vi "Oclaro_FB_INJ_ActiveSampling.vi"(1 "Resistance (k Ohms)":dbl=10.0) -> ()   [LabVIEW 2014]
doc: "Use this template to measure or generate signals using the DAQ Assistant Express VI and NI-DAQmx. Double click the DAQ Assistant Express VI to launch a configuration wizard which steps you through configuring a measurement or generation.\n\nNote: You must have an NI-DAQmx compatible device installed to use this Express VI. Refer to the DAQ Quick Start Guide for NI-DAQ 7.0 for a list of compatible devices."
uses:
  <vilib>/addons/zeromq/socket_type.ctl
  Instance           8 18Saved   INJ FB Map .vi
  <instrlib>/Tektronix 7000 Series/Public/Data/Read (Single Waveform).vi
  <instrlib>/Tektronix 7000 Series/Tektronix 7000 Series.lvlib
  <vilib>/addons/zeromq/zeromq.lvlib
  <vilib>/addons/zeromq/zmq_context.lvclass
  <vilib>/addons/zeromq/zmq_socket.lvclass
panel:
  in  "AOM Channel":bool
  out "Status":string="Complete"
  out "Start time":timestamp=timestamp(3523998390.26649 s since 1904-01-01)
  in  "Current Source Address":refnum<visa-resource-name>="GPIB0::3::INSTR"
  in  "TEC Address":refnum<visa-resource-name>="GPIB0::3::INSTR"
  in  "Channel (0: Channel 1)":u16(ring)=3 format="%#_5f" items=["Channel 1", "Channel 2", "Channel 3", "Channel 4", "Math 1", "Math 2", "Math 3", "Math 4", "Reference 1", "Reference 2", "Reference 3", "Reference 4"]
  out "Total Time (hrs)":dbl=0.15259278178215027
  out "Finish time":timestamp=timestamp(3523998939.6005044 s since 1904-01-01)
  in  "Tek Scope Address":refnum<visa-resource-name>="GPIB0::4::INSTR"
  in  "Time to wait for TEC (sec)":dbl=10.0 caption="Delay Time (s)"
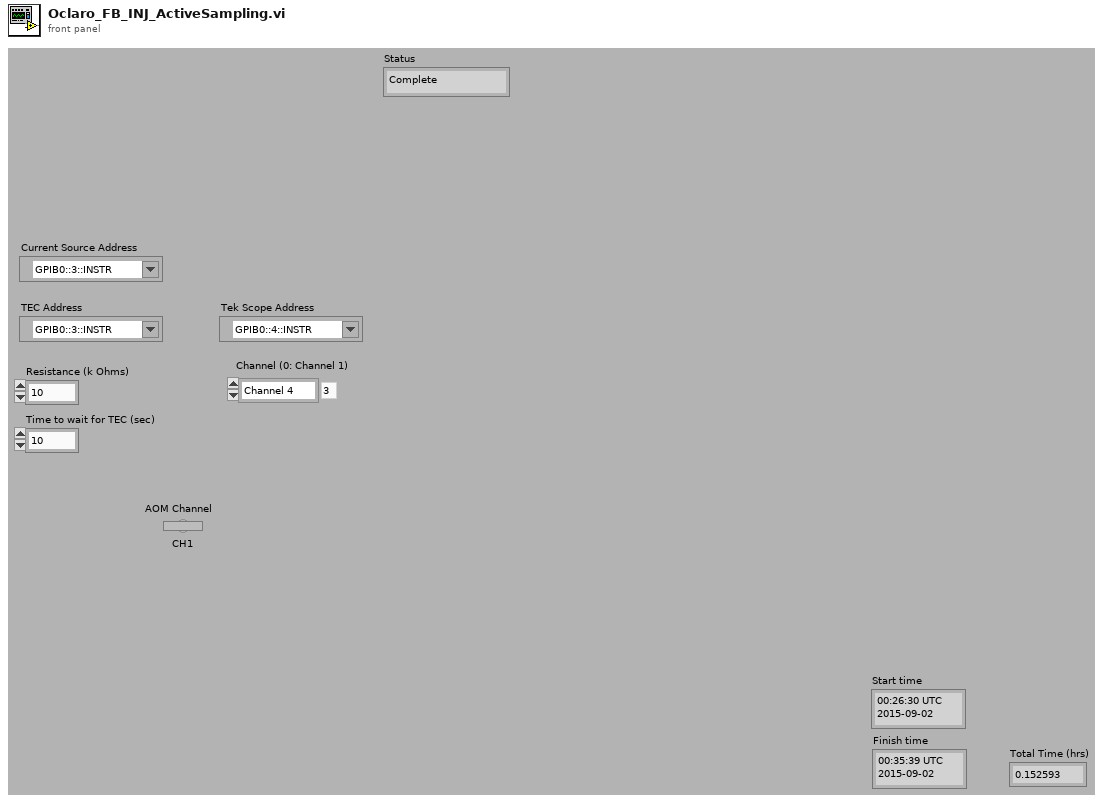
[diagram p1: front panel]
types:
  T1 = typedef "zeromq.lvlib/socket_type.ctl" = enum8{"ZMQ_PAIR", "ZMQ_PUB", "ZMQ_SUB", "ZMQ_REQ", "ZMQ_REP", "ZMQ_DEALER", "ZMQ_ROUTER", "ZMQ_PULL", "ZMQ_PUSH", "ZMQ_XPUB", "ZMQ_XSUB"}
  T2 = enum16{"big-endian, network order", "native, host order", "little-endian"}
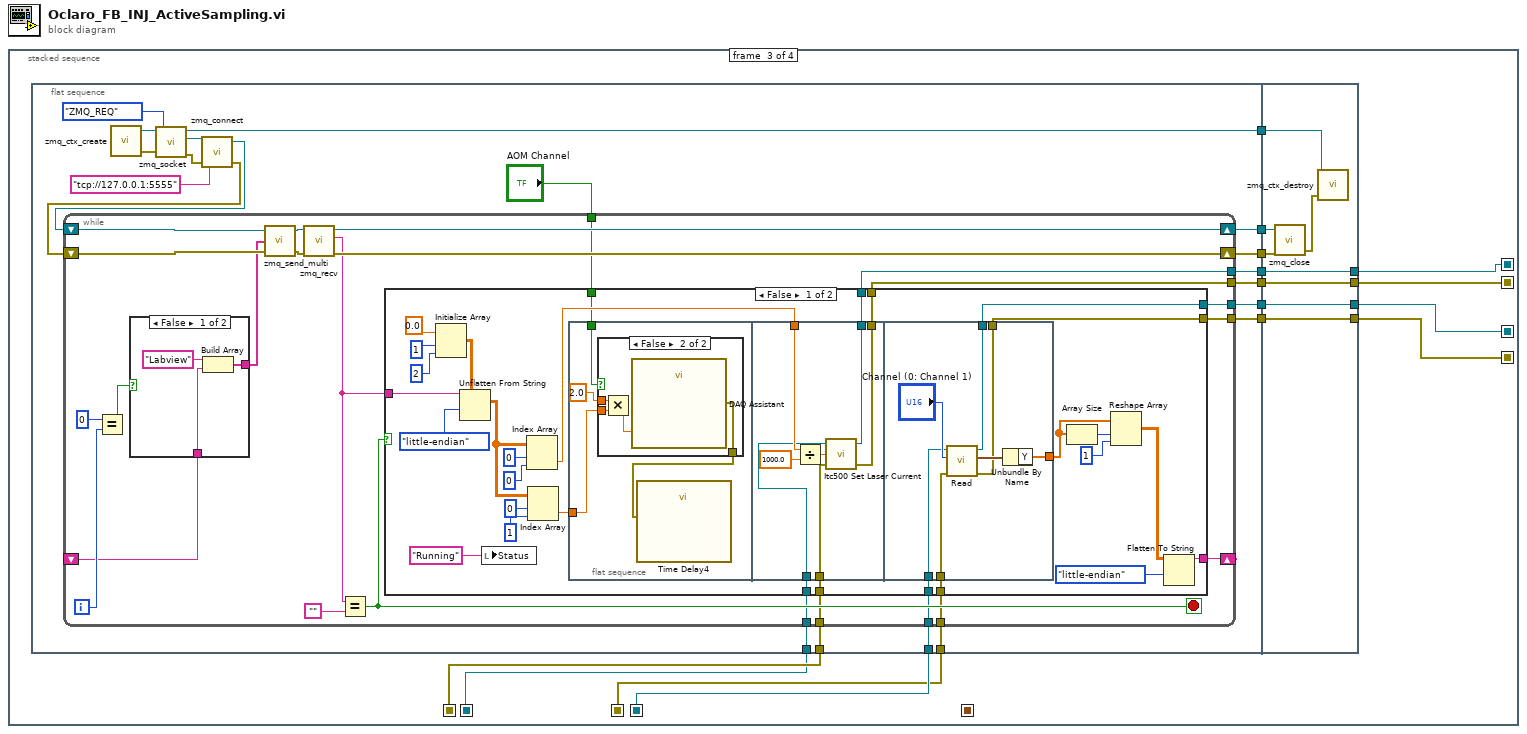
[diagram p0: block diagram]
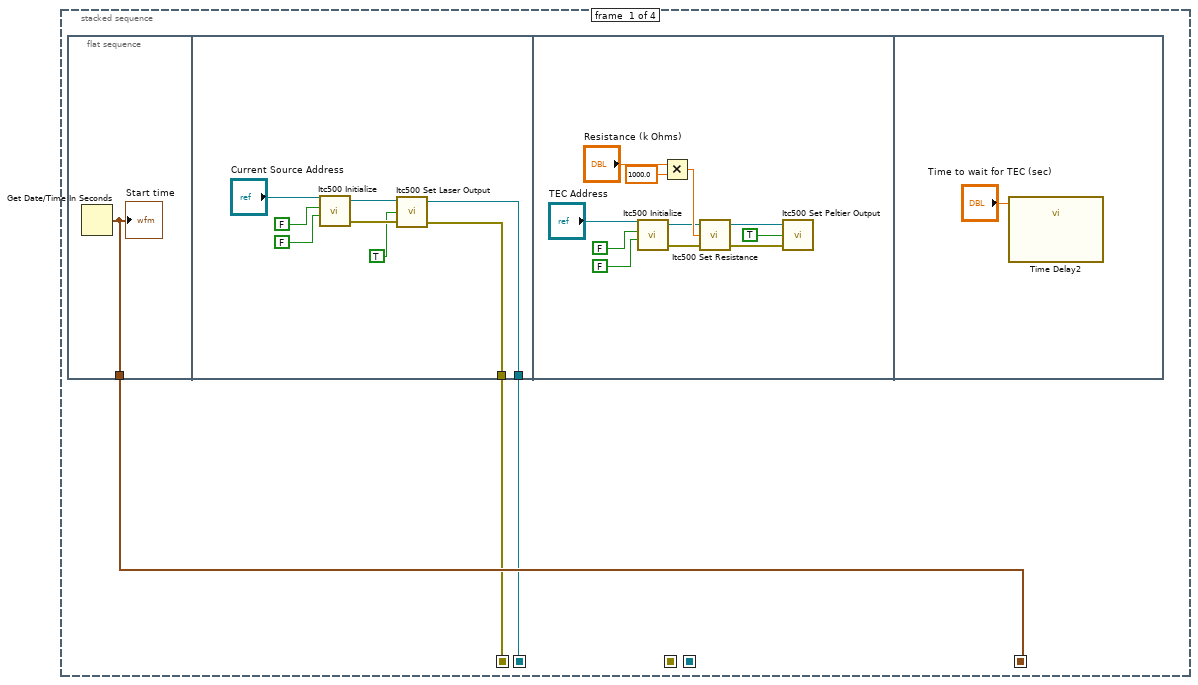
[diagram p2: hidden frame]
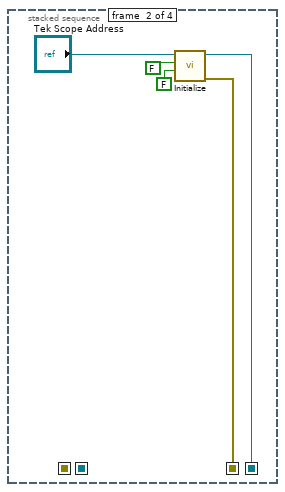
[diagram p3: hidden frame]
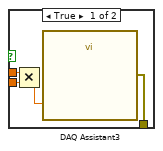
[diagram p4: hidden frame]
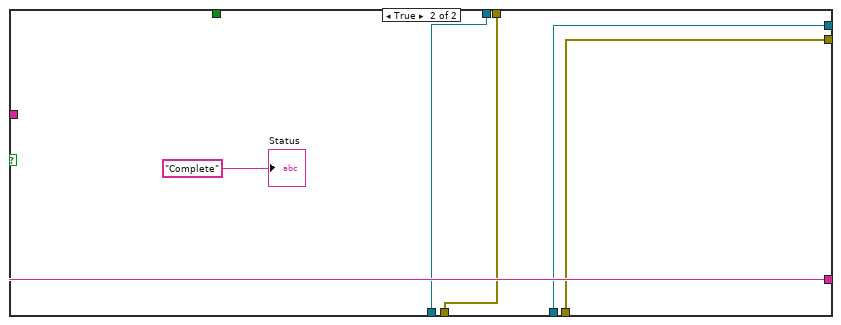
[diagram p5: hidden frame]
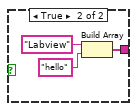
[diagram p6: hidden frame]
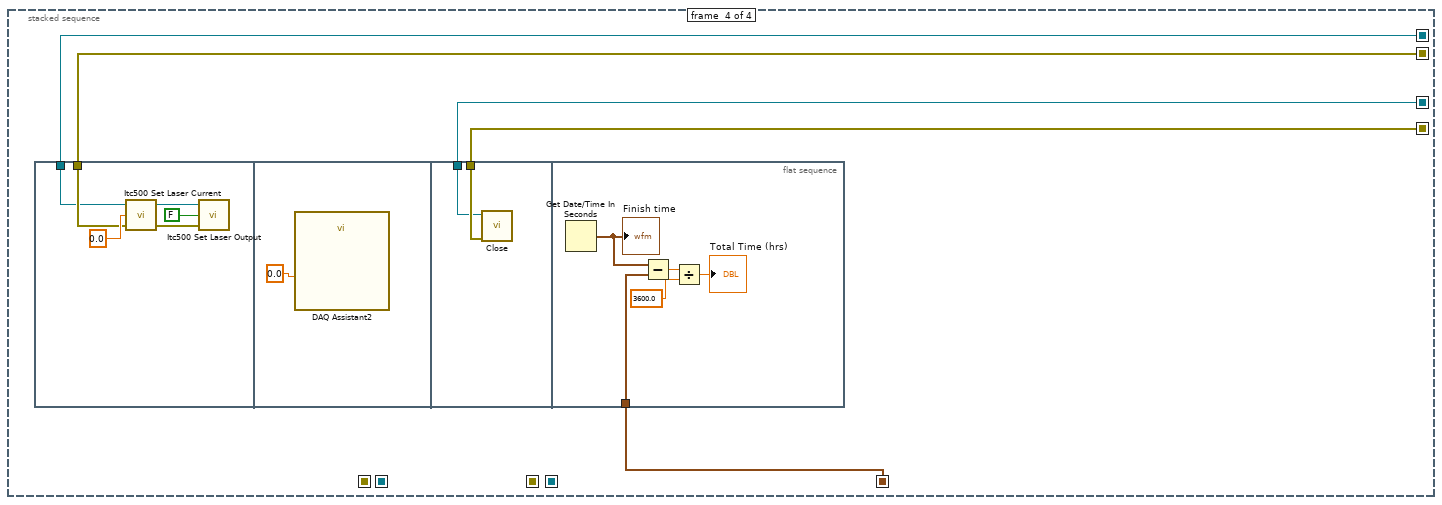
[diagram p7: hidden frame]
diagram:
  n1 = stacked-sequence {
    seq-local: [_ w25 _ _] -> [_ _ w38 _]
    seq-local: [_ w26 _ _] -> [_ _ w39 _]
    seq-local: [_ _ w30 _] -> [_ _ _ w167]
    seq-local: [_ _ w32 _] -> [_ _ _ w168]
    seq-local: [w3 _ _ _] -> [_ _ _ w164]
    seq-local: [_ _ w34 _] -> [_ _ _ w165]
    seq-local: [_ _ w36 _] -> [_ _ _ w166]
    seq-local: [w1 _ _ _] -> [_ _ w40 _]
    seq-local: [w2 _ _ _] -> [_ _ w41 _]
    frame #0 {
      n2 = flat-sequence {
        tunnel: [w4] -> w3
        tunnel: [w6] -> w2
        tunnel: [w5] -> w1
        frame #0 {
          n3 = Get Date/Time In Seconds() -> (seconds since 1Jan1904=w4:timestamp)
          "Start time" <- w4
        }
        frame #1 {
          n4 = call <instrlib>:"Itc500 Initialize.vi"("reset device"=FALSE, "id query"=FALSE, "resource name"="Current Source Address") -> ("error out"=w12:errorcluster, "instrument handle"=w11:refnum<visa-resource-name>)  [unwired: 1 in, 1 out]
          n5 = call <instrlib>:"Itc500 Set Laser Output.vi"("error in (no error)"=w12, "output"=TRUE, "instrument handle"=w11) -> ("error out"=w6:errorcluster, "instrument handle out"=w5:refnum<visa-resource-name>)  [unwired: 1 out]
        }
        frame #2 {
          n6 = call <instrlib>:"Itc500 Initialize.vi"("reset device"=FALSE, "id query"=FALSE, "resource name"="TEC Address") -> ("error out"=w19:errorcluster, "instrument handle"=w18:refnum<visa-resource-name>)  [unwired: 1 in, 1 out]
          n7 = Multiply(x="Resistance (k Ohms)", y=1000.0) -> (x*y=w22:dbl)
          n8 = call <instrlib>:"Itc500 Set Resistance.vi"("error in (no error)"=w19, "resistance"=w22, "instrument handle"=w18) -> ("error out"=w16:errorcluster, "instrument handle out"=w15:refnum<visa-resource-name>)  [unwired: 1 out]
          n9 = call <instrlib>:"Itc500 Set Peltier Output.vi"("error in (no error)"=w16, "output"=TRUE, "instrument handle"=w15) -> ()  [unwired: 3 out]
        }
        frame #3 {
          n10 = call "Time Delay2"("Delay Time (s)"="Time to wait for TEC (sec)") -> ()  [unwired: 10 in, 1 out]
        }
      }
    }
    frame #1 {
      n11 = call <instrlib>:"Initialize.vi"("Reset? ( Yes)"=FALSE ("Reset (T: Reset)"), "ID Query? ( Yes)"=FALSE ("Reset (T: Reset)"), "VISA resource name"="Tek Scope Address") -> ("error out"=w25:errorcluster, "VISA resource name out"=w26:refnum<visa-resource-name>)  [unwired: 7 in]
    }
    frame #2 {
      n12 = flat-sequence {
        tunnel: [w60] -> w44
        tunnel: [w54] -> w43
        tunnel: [w55] -> w42
        tunnel: w41 -> [w53]
        tunnel: w40 -> [w52]
        tunnel: w39 -> [w51]
        tunnel: w38 -> [w50]
        tunnel: [w49] -> w37
        tunnel: [w48] -> w35
        tunnel: [w47] -> w33
        tunnel: [w46] -> w31
        tunnel: w44 -> [w163]
        tunnel: w43 -> [w161]
        tunnel: w42 -> [w160]
        tunnel: [w159] -> w36
        tunnel: w37 -> [w159]
        tunnel: [w158] -> w34
        tunnel: w35 -> [w158]
        tunnel: [w157] -> w32
        tunnel: w33 -> [w157]
        tunnel: [w156] -> w30
        tunnel: w31 -> [w156]
        frame #0 {
          n13 = call <vilib>:"zmq_ctx_create.vi"() -> ("error out"=w59:errorcluster, "context out"=w64:refnum<class "zmq_context.lvclass">)  [unwired: 4 in]
          n14 = call <vilib>:"zmq_socket.vi"("error in"=w59, "socket type"=socket_type."ZMQ_REQ", "context in"=w64) -> ("error out"=w63:errorcluster, "socket out"=w62:refnum<class "zmq_socket.lvclass">, "context out"=w60:refnum<class "zmq_context.lvclass">)  [unwired: 2 in]
          n15 = call <vilib>:"zmq_connect.vi"("error in"=w63, "endpoint"="tcp://127.0.0.1:5555", "socket in"=w62) -> ("error out"=w56:errorcluster, "socket out"=w61:refnum<class "zmq_socket.lvclass">)  [unwired: 1 in]
          n16 = while {
            shift-right: [w83] -> w54
            shift-left: w61 -> [w88]
            shift-right: [w84] -> w55
            shift-left: w56 -> [w87]
            shift-right: [w82] -> _
            shift-left: _ -> [w78]
            tunnel: w53 -> [w73]
            tunnel: w52 -> [w72]
            tunnel: w51 -> [w71]
            tunnel: w50 -> [w70]
            tunnel: [w69] -> w49
            tunnel: [w68] -> w48
            tunnel: [w67] -> w47
            tunnel: [w66] -> w46
            tunnel: "AOM Channel" -> [w65]
            i -> [w81]
            stop <- w75 stop-if-true
            n17 = Equal?(x=0, y=w81) -> (x = y?=w79:bool)
            n18 = case shown="False" w79 {
              tunnel: [w151 w155] -> w74
              tunnel: w78 -> [w150 _]
              frame False {
                n19 = Build Array("Labview", w150) -> (w151:string[])
              }
              frame True {
                n20 = Build Array("Labview", "hello" ("element")) -> (w155:string[])
              }
            }
            n21 = call <vilib>:"zmq_send_multi.vi"("error in"=w87, "parts"=w74, "socket in"=w88) -> ("error out"=w85:errorcluster, "socket out"=w86:refnum<class "zmq_socket.lvclass">)  [unwired: 1 in]
            n22 = call <vilib>:"zmq_recv.vi"("error in"=w85, "socket in"=w86) -> ("error out"=w84:errorcluster, "data"=w76:string, "socket out"=w83:refnum<class "zmq_socket.lvclass">)  [unwired: 3 in, 2 out]
            n23 = Equal?(x=w76, y="") -> (x = y?=w75:bool)
            n24 = case shown="False" w75 {
              tunnel: [w106 w149] -> w82
              tunnel: w76 -> [w105 w149]
              tunnel: w73 -> [w97 w146]
              tunnel: w72 -> [w96 w147]
              tunnel: w71 -> [w95 w145]
              tunnel: w70 -> [w94 w144]
              tunnel: [w93 w144] -> w69
              tunnel: [w92 w145] -> w68
              tunnel: [w91 w147] -> w66
              tunnel: [w90 w146] -> w67
              tunnel: w65 -> [w89 _]
              frame False {
                n25 = Initialize Array(0.0, 1 ("dimension size"), 2 ("dimension size")) -> (w113:dbl[][])
                n26 = Unflatten From String(type=w113, binary string=w105, byte order (0:big-endian, network order)=T2."little-endian") -> (value=w110:dbl[][])  [unwired: 2 in, 2 out]
                n27 = local write "Status"("Running" ("Status")) -> ()
                n28 = Index Array(array=w110, index (row)=0 ("disabled index (row)"), index (col)=0 ("disabled index (col)")) -> (element=w102:dbl)
                n29 = Index Array(array=w110, index (row)=0 ("disabled index (row)"), index (col)=1 ("disabled index (col)")) -> (element=w103:dbl)
                n30 = flat-sequence {
                  tunnel: w103 -> [w119]
                  tunnel: w89 -> [w118]
                  tunnel: w102 -> [w134]
                  tunnel: w97 -> [w133]
                  tunnel: w96 -> [w132]
                  tunnel: [w131] -> w91
                  tunnel: [w130] -> w90
                  tunnel: [w141] -> w100
                  tunnel: w95 -> [w140]
                  tunnel: w94 -> [w139]
                  tunnel: [w138] -> w92
                  tunnel: [w137] -> w93
                  frame #0 {
                    n31 = case shown="False" w118 {
                      tunnel: 2.0 ("x") -> [w124 w128]
                      tunnel: [w123 w127] -> w120
                      tunnel: w119 -> [w122 w126]
                      frame True {
                        n32 = Multiply(x=w124, y=w122) -> (x*y=w125:dbl)
                        n33 = call "DAQ Assistant3"("data"=w125) -> ("error out"=w123:errorcluster)  [unwired: 17 in, 1 out]
                      }
                      frame False {
                        n34 = Multiply(x=w128, y=w126) -> (x*y=w129:dbl)
                        n35 = call "DAQ Assistant"("data"=w129) -> ("error out"=w127:errorcluster)  [unwired: 17 in, 1 out]
                      }
                    }
                    n36 = call "Time Delay4"("error in (no error)"=w120) -> ()  [unwired: 10 in, 1 out]
                  }
                  frame #1 {
                    n37 = Divide(x=w134, y=1000.0) -> (x/y=w135:dbl)
                    n38 = call <instrlib>:"Itc500 Set Laser Current.vi"("error in (no error)"=w133, "current"=w135, "instrument handle"=w132) -> ("error out"=w130:errorcluster, "instrument handle out"=w131:refnum<visa-resource-name>)  [unwired: 1 out]
                  }
                  frame #2 {
                    n39 = call-poly <instrlib>:"Read.vi"("error in (no error)"=w139, "Channel (0: Channel 1)"="Channel (0: Channel 1)", "VISA resource name"=w140) -> ("error out"=w137:errorcluster, "Waveform Data"=w143:waveform(dbl), "VISA resource name out"=w138:refnum<visa-resource-name>)  [unwired: 6 in]
                    n40 = Unbundle By Name(w143) -> ("Y"=w141:dbl[])
                  }
                }
                n41 = Array Size(array=w100) -> (size(s)=w99:i32)
                n42 = Reshape Array(w100, w99, 1 ("dimension size")) -> (w98:dbl[][])
                n43 = Flatten To String(anything=w98, byte order (0:big-endian, network order)=T2."little-endian") -> (data string=w106:string)  [unwired: 2 in, 2 out]
              }
              frame True {
                "Status" <- "Complete"
              }
            }
          }
        }
        frame #1 {
          n44 = call <vilib>:"zmq_close.vi"("error in"=w160, "socket"=w161) -> ("error out"=w162:errorcluster)  [unwired: 3 in]
          n45 = call <vilib>:"zmq_ctx_destroy.vi"("error in"=w162, "context in"=w163) -> ()  [unwired: 3 in, 1 out]
        }
      }
    }
    frame #3 {
      n46 = flat-sequence {
        tunnel: w168 -> [w170]
        tunnel: w167 -> [w169]
        tunnel: w166 -> [w177]
        tunnel: w165 -> [w176]
        tunnel: w164 -> [w178]
        frame #0 {
          n47 = call <instrlib>:"Itc500 Set Laser Current.vi"("error in (no error)"=w170, "current"=0.0, "instrument handle"=w169) -> ("error out"=w173:errorcluster, "instrument handle out"=w172:refnum<visa-resource-name>)  [unwired: 1 out]
          n48 = call <instrlib>:"Itc500 Set Laser Output.vi"("error in (no error)"=w173, "output"=FALSE, "instrument handle"=w172) -> ()  [unwired: 3 out]
        }
        frame #1 {
          n49 = call "DAQ Assistant2"("data"=0.0) -> ()  [unwired: 17 in, 2 out]
        }
        frame #2 {
          n50 = call <instrlib>:"Close.vi"("error in (no error)"=w177, "VISA resource name"=w176) -> ()  [unwired: 9 in, 1 out]
        }
        frame #3 {
          n51 = Get Date/Time In Seconds() -> (seconds since 1Jan1904=w179:timestamp)
          "Finish time" <- w179
          n52 = Subtract(x=w179, y=w178) -> (x-y=w181:dbl)
          n53 = Divide(x=w181, y=3600.0) -> (x/y=→"Total Time (hrs)":dbl)
        }
      }
    }
  }
